vi "Get SubpanelVI Info.vi"(8 "error in (no error)":errorcluster, 11 "VacuumLines Configuration in":refnum<class "VacuumLines Configuration.lvclass">) -> (0 "error out":errorcluster, 1 "Array of Subpanel VI data":T1[](array[typedef]), 2 "Array of Category string":string[](array[string]), 3 "VacuumLines Configuration out":refnum<class "VacuumLines Configuration.lvclass">)   [LabVIEW 2016, in "Hardware.lvlib" / "VacuumLine.lvlib" / "VacuumLines Configuration.lvclass"]
uses:
  <userlib>/Common Components/Hardware/Abstract System/VacuumLine/VacuumLines Configuration/VacuumLines Configuration.lvclass
  <userlib>/Configuration Dialog Actor/Methods/Data Retrieved by Lookup Table.ctl
  <userlib>/Configuration Dialog Actor/Configuration.lvclass
  <userlib>/Common Components/Hardware/Abstract System/VacuumLine/VacuumLines Configuration/Config Conflict Zones.vi
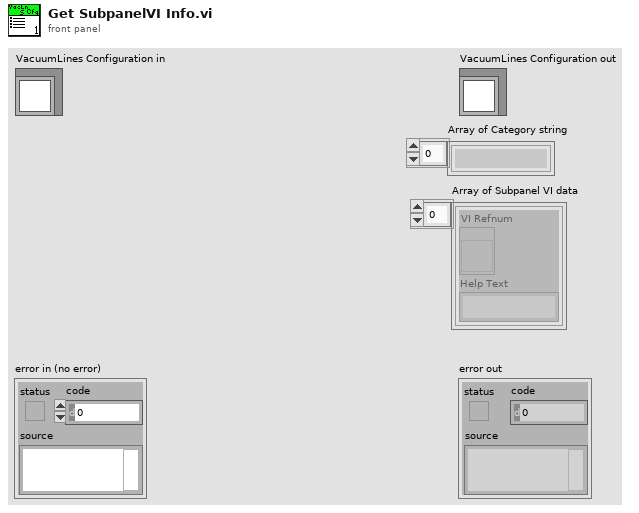
[diagram p1: front panel]
types:
  T1 = typedef "Configuration.lvlib/Configuration.lvclass/Data Retrieved by Lookup Table.ctl" = cluster{"VI Refnum":refnum<vi>, "Help Text":string}
  T2 = cluster{"Conflict Zones":string, "More Valves":string, "Pressure Display":string, "Temperature":string}
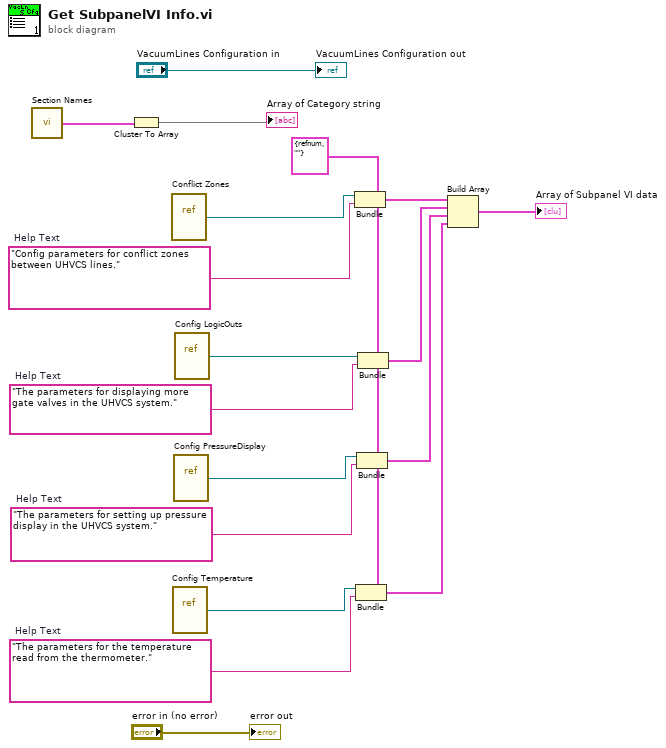
[diagram p0: block diagram]
diagram:
  w3 = "Config parameters for conflict zones between UHVCS lines."  # Help Text
  w6 = "The parameters for the temperature read from the thermometer."  # Help Text
  w9 = "The parameters for setting up pressure display in the UHVCS system."  # Help Text
  w14 = "The parameters for displaying more gate valves in the UHVCS system."  # Help Text
  w2 = T1 {"VI Refnum"=refnum, "Help Text"=""} ("output cluster")
  n1 = call <userlib>:"Section Names.vi"() -> ("Cluster"=w12:T2)
  n2 = Cluster To Array(cluster=w12) -> (array=→"Array of Category string":string[])
  n3 = vi-ref "Conflict Zones.vi"() -> (w4:refnum<vi>)
  n4 = vi-ref <userlib>:"Config Temperature.vi"() -> (w7:refnum<vi>)
  n5 = vi-ref <userlib>:"Config PressureDisplay.vi"() -> (w10:refnum<vi>)
  n6 = vi-ref <userlib>:"Config LogicOuts.vi"() -> (w15:refnum<vi>)
  n7 = Bundle(cluster=w2, "VI Refnum"=w4, "Help Text"=w3) -> (w1:T1)
  n8 = Bundle(cluster=w2, "VI Refnum"=w7, "Help Text"=w6) -> (w5:T1)
  n9 = Bundle(cluster=w2, "VI Refnum"=w10, "Help Text"=w9) -> (w8:T1)
  n10 = Bundle(cluster=w2, "VI Refnum"=w15, "Help Text"=w14) -> (w16:T1)
  n11 = Build Array(w1, w16, w8, w5) -> (→"Array of Subpanel VI data":T1[])
  "error out" <- "error in (no error)"
  "VacuumLines Configuration out" <- "VacuumLines Configuration in"
